vi "lvssh2_session_callback_register_send_64.vi"(11 "send":refnum<vi>) -> (0 "error out":errorcluster, 2 "stop event":refnum<user-event>, 3 "user event":refnum<user-event>)   [LabVIEW 2017, in "libssh2.lvlib"]
uses:
  libssh2.lvlib
  lvssh2_session_callback_send_function_input_args_64.ctl
  lvssh2_session_callback_send_handler_64.vi
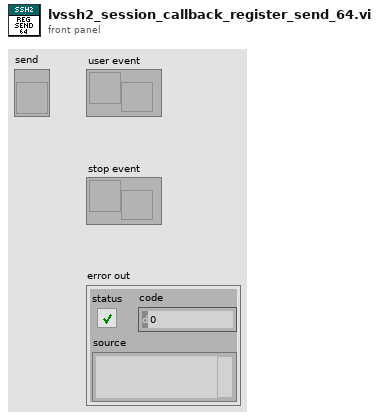
[diagram p1: front panel]
types:
  T1 = typedef "libssh2.lvlib/lvssh2_session_callback_send_function_input_args_64.ctl" = cluster{"*socket":u64, "buffer":u8[], "flags":i32, "<padding>":i32, "*bytes_send":u64, "completion":u64}
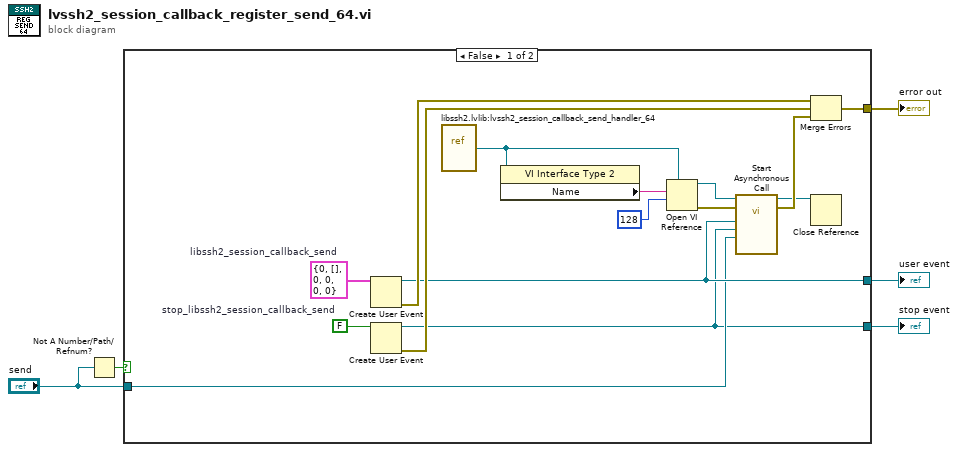
[diagram p0: block diagram]
diagram:
  n1 = Not A Number/Path/Refnum?(number/path/refnum="send") -> (NaN/Path/Refnum?=w2:bool)
  n2 = case shown="False" w2 {
    tunnel: [w11 _] -> w5
    tunnel: [w20 _] -> w4
    tunnel: "send" -> [w9 _]
    tunnel: [w7 _] -> w1
    frame False {
      w17 = FALSE  # stop_libssh2_session_callback_send
      w19 = T1 {"*socket"=0, "buffer"=[], "flags"=0, "<padding>"=0, "*bytes_send"=0, "completion"=0}  # libssh2_session_callback_send
      n3 = Create User Event(user event datatype=w19) -> (user event=w11:refnum<user-event>, error out=w18:errorcluster)  [unwired: 1 in]
      n4 = Create User Event(user event datatype=w17) -> (user event=w7:refnum<user-event>, error out=w16:errorcluster)  [unwired: 1 in]
      n5 = vi-ref "libssh2.lvlib:lvssh2_session_callback_send_handler_64.vi"() -> ("vi reference"=w10:refnum<vi>)
      n6 = property class="VI Interface Type 2"(reference=w10) -> ("Name"=w13:string)  [unwired: 1 in, 2 out]
      n7 = Open VI Reference(type specifier VI Refnum (for type only)=w10, vi path=w13, options=128) -> (vi reference=w15:refnum<vi>, error out=w14:errorcluster)  [unwired: 3 in]
      n8 = call-by-ref "Start Asynchronous Call"(reference=w15, error in=w14, "lvssh2_session_callback_send"=w9, "Stop Event Ref"=w7, "User Event Ref"=w11) -> (reference out=w6:refnum<vi>, error out=w8:errorcluster)  [unwired: 9 in]
      n9 = Merge Errors(w18, w16, w8) -> (w20:errorcluster)
      n10 = Close Reference(reference=w6) -> ()  [unwired: 1 in, 1 out]
    }
    frame True {
    }
  }
  "user event" <- w5
  "error out" <- w4
  "stop event" <- w1
